vi "Caller.vi"(0 "Divide in":refnum<class "Divide.lvclass">, 2 "DVR In":refnum<data-value>, 5 "Sub Panel":refnum<vi>, 7 "State":refnum<user-event>, 9 "Class Data":refnum<user-event>, 11 "Error In":errorcluster) -> (4 "Divide out":refnum<class "Divide.lvclass">, 15 "Error Out":errorcluster)   [LabVIEW 2019, in "Divide.lvclass"]
doc: "The VI asynchronously calls the Operation UI method of the division operation."
uses:
  Divide.lvclass
  Operation UI.vi
  Arithemtic Operation/Arithemetic Operation.lvclass
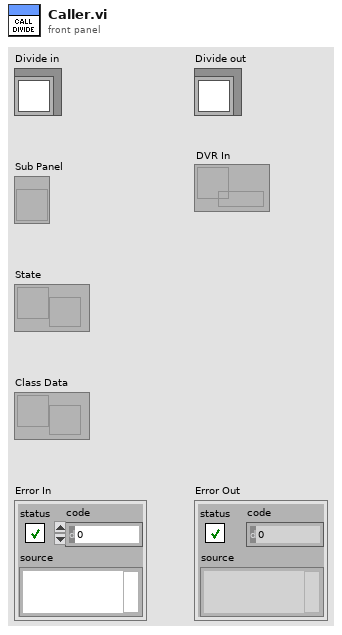
[diagram p1: front panel]
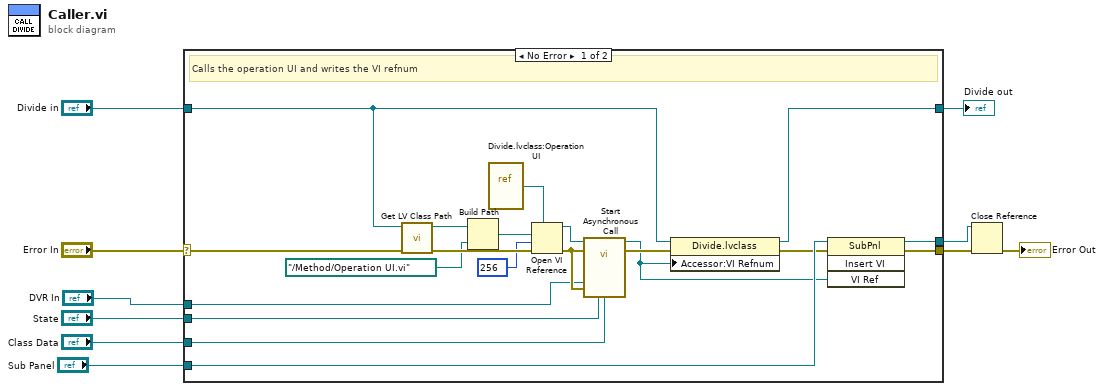
[diagram p0: block diagram]
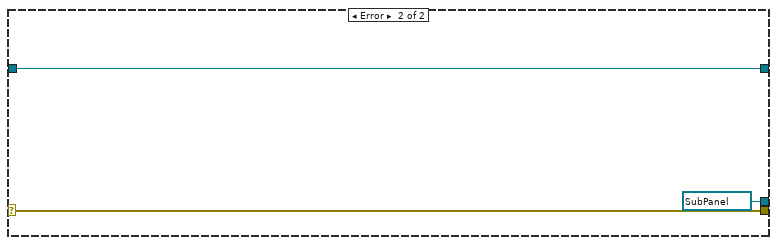
[diagram p2: hidden frame]
diagram:
  n1 = case shown="No Error" "Error In" {
    selector: "Error In" -> [w23 w33]
    tunnel: [w22 w33] -> w9
    tunnel: [w18 w32] -> w7
    tunnel: "Divide in" -> [w16 w32]
    tunnel: "State" -> [w13 _]
    tunnel: "Class Data" -> [w12 _]
    tunnel: "Sub Panel" -> [w21 _]
    tunnel: [w17 refnum<vi> refnum ("Sub Panel")] -> w2
    tunnel: "DVR In" -> [w11 _]
    frame No Error {
      # "Calls the operation UI and writes the VI refnum"
      n2 = call <vilib>:"Get LV Class Path.vi"("error in (no error)"=w23, "object"=w16) -> ("error out"=w30:errorcluster, "class path"=w29:path)  [unwired: 8 in]
      n3 = Build Path(base path=w29, name or relative path=path "../Method/Operation UI.vi") -> (appended path=w15:path)
      n4 = vi-ref "Divide.lvclass:Operation UI.vi"() -> (w24:refnum<vi>)
      n5 = Open VI Reference(type specifier VI Refnum (for type only)=w24, vi path=w15, options=256, error in (no error)=w30) -> (vi reference=w27:refnum<vi>, error out=w14:errorcluster)  [unwired: 2 in]
      n6 = call-by-ref "Start Asynchronous Call"(reference=w27, error in=w14, "DVR In"=w11, "Error In"=w14, "Stop"=w13, "Class Data"=w12) -> (reference out=w19:refnum<vi>, error out=w26:errorcluster)  [unwired: 9 in, 3 out]
      n7 = property class="Divide.lvclass"(reference=w16, error in=w26, "Accessor:VI Refnum"=w19) -> (reference out=w18:refnum<class "Divide.lvclass">, error out=w20:errorcluster)
      n8 = invoke on="Invoke Node" class="SubPnl" method="Insert VI"(reference=w21, error in=w20, "VI Ref"=w19) -> (reference out=w17:refnum<vi>, error out=w22:errorcluster)  [unwired: 1 in, 2 out]
    }
    frame Error {
    }
  }
  "Divide out" <- w7
  n9 = Close Reference(reference=w2, error in (no error)=w9) -> (error out=→"Error Out":errorcluster)
